vi "Enter.vi"(8 "error in (no error)":errorcluster, 11 "Door in":refnum<class "Door.lvclass">) -> (0 "error out":errorcluster, 3 "Door out":refnum<class "Door.lvclass">)   [LabVIEW 2016, in "Door.lvclass"]
uses:
  Door.lvclass
  MapSite/MapSite.lvclass
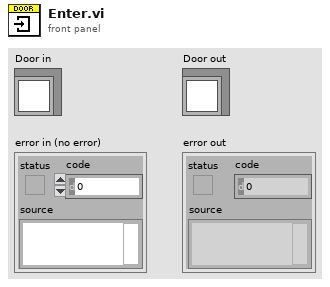
[diagram p1: front panel]
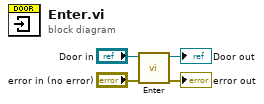
[diagram p0: block diagram]
diagram:
  n1 = call-parent "Enter.vi"("error in (no error)"="error in (no error)", "MapSite in"="Door in") -> ("error out"=→"error out":errorcluster, "MapSite out"=→"Door out":refnum<class "Door.lvclass">)  [unwired: 8 in]
